vi "get_codecs.vi"() -> ()   [LabVIEW 2017]
panel:
  out "Codec Names":string[](array[string])
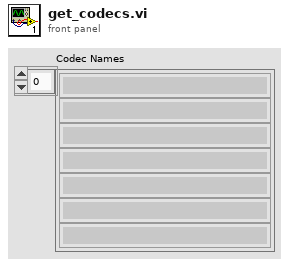
[diagram p1: front panel]
types:
  T1 = typedef "Image Type" = u32
  T2 = typedef "IMAQ Image.ctl" = refnum<image>
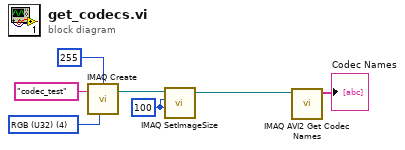
[diagram p0: block diagram]
diagram:
  w3 = 100 ("X Resolution")
  w7 = T1 4 items=["Grayscale (U8)", "Grayscale (I16)", "Grayscale (SGL)", "Complex (CSG)", "RGB (U32)", "HSL (U32)", "RGB (U64)", "Grayscale (U16)"] ("Image Type")
  n1 = call "IMAQ Create"("Border Size"=255, "Image Name"="codec_test", "Image Type"=w7) -> ("New Image"=w2:T2)  [unwired: 2 in, 1 out]
  n2 = call "IMAQ SetImageSize"("Y Resolution"=w3, "X Resolution"=w3, "Image"=w2) -> ("Image Out"=w1:T2)  [unwired: 2 in, 1 out]
  n3 = call "IMAQ AVI2 Get Codec Names"("Image"=w1) -> ("Codec Names"=→"Codec Names":string[])  [unwired: 9 in, 1 out]
